vi "Define Channel Count.vi"(8 "error in":errorcluster, 11 "NI 9422 in":refnum<class "NI 9422.lvclass">) -> (0 "error out":errorcluster, 3 "NI 9422 out":refnum<class "NI 9422.lvclass">)   [LabVIEW 2020, in "Scan Engine Scripting.lvlib" / "NI 9422.lvclass"]
uses:
  NI 9422.lvclass
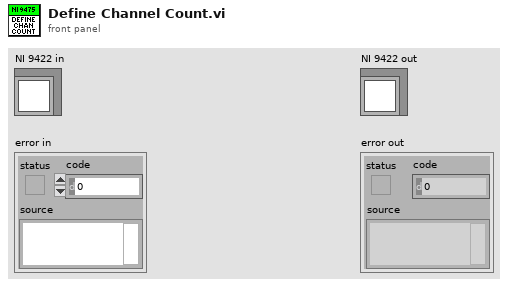
[diagram p1: front panel]
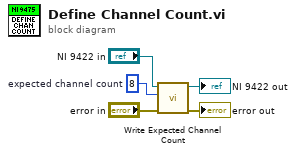
[diagram p0: block diagram]
diagram:
  w3 = u8 8  # expected channel count
  n1 = call-dynamic "Write Expected Channel Count.vi"("error in"="error in", "expected channel count"=w3, "module in"="NI 9422 in") -> ("error out"=→"error out":errorcluster, "module out"=→"NI 9422 out":refnum<class "NI 9422.lvclass">)  [unwired: 7 in]
